vi "Parse for Instrument Name.vi"(9 "Instrument Name":string, 10 "Message In":T1, 11 "UI In":refnum<queue>) -> (2 "Message Out":T1)   [LabVIEW 2014, in "Flicker.lvlib" / "Flicker Message Queue.lvlib"]
uses:
  Message Cluster.ctl
  <vilib>/regexp/Match Regular Expression.xnode
  Flicker Message Queue.lvlib
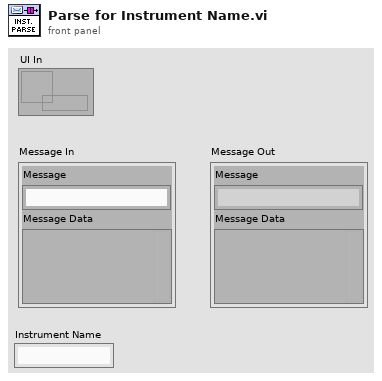
[diagram p1: front panel]
types:
  T1 = typedef "Flicker.lvlib/Flicker Message Queue.lvlib/Message Cluster.ctl" = cluster{"Message":string, "Message Data":variant}
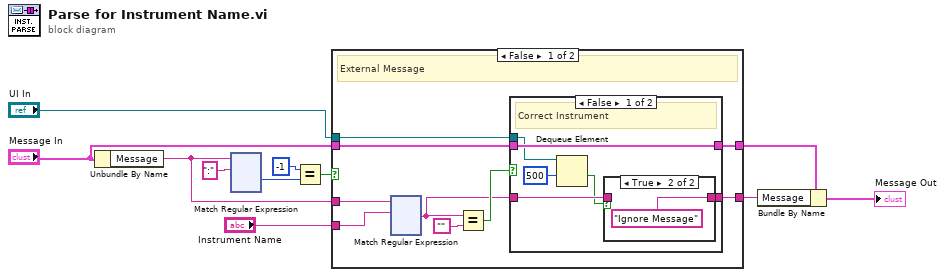
[diagram p0: block diagram]
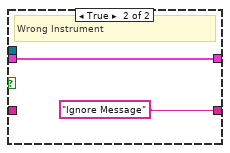
[diagram p3: hidden frame]
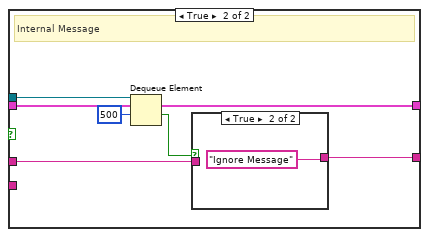
[diagram p4: hidden frame]
diagram:
  n1 = Unbundle By Name("Message In") -> ("Message"=w6:string)
  n2 = xnode "Match Regular Expression"("input string"=w6, "regular expression"=":") -> ("offset past match"=w10:i32)  [unwired: 4 in, 4 out]
  n3 = Equal?(x=-1, y=w10) -> (x = y?=w8:bool)
  n4 = case shown="False" w8 {
    tunnel: [w15 w145] -> w5
    tunnel: "Instrument Name" -> [w20 _]
    tunnel: w6 -> [w18 w146]
    tunnel: "UI In" -> [w14 w149]
    tunnel: "Message In" -> [w13 w150]
    tunnel: [w12 w150] -> w4
    frame False {
      # "External Message"
      n5 = xnode "Match Regular Expression"("input string"=w18, "regular expression"=w20) -> ("after match"=w16:string)  [unwired: 4 in, 4 out]
      n6 = Equal?(x=w16, y="") -> (x = y?=w17:bool)
      n7 = case shown="False" w17 {
        tunnel: w16 -> [w23 _]
        tunnel: [w22 "Ignore Message" ("t")] -> w15
        tunnel: w14 -> [w25 _]
        tunnel: w13 -> [w26 w29]
        tunnel: [w26 w29] -> w12
        frame False {
          # "Correct Instrument"
          n8 = Dequeue Element(queue=w25, timeout in ms (-1)=500) -> (timed out?=w21:bool)  [unwired: 1 in, 3 out]
          n9 = case shown="True" w21 {
            tunnel: w23 -> [w27 _]
            tunnel: [w27 "Ignore Message"] -> w22
            frame False {
            }
            frame True {
            }
          }
        }
        frame True {
          # "Wrong Instrument"
        }
      }
    }
    frame True {
      # "Internal Message"
      n10 = Dequeue Element(queue=w149, timeout in ms (-1)=500) -> (timed out?=w147:bool)  [unwired: 1 in, 3 out]
      n11 = case shown="True" w147 {
        tunnel: w146 -> [w151 _]
        tunnel: [w151 "Ignore Message"] -> w145
        frame False {
        }
        frame True {
        }
      }
    }
  }
  n12 = Bundle By Name(cluster=w4, "Message"=w5) -> (→"Message Out":T1)
